vi "Poly-fit.vi"(3 "QPD signal (V)":dbl[](array[numeric]), 5 "stage position (um)":dbl[](array[numeric])) -> (1 "Polynomial Coefficients":dbl[](array[numeric]), 2 "Best stage position":dbl[](array[numeric]))   [LabVIEW 2014]
uses:
  <vilib>/Analysis/NI_AALPro.lvlib
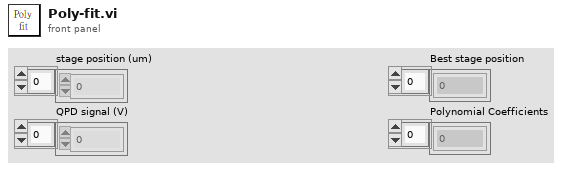
[diagram p1: front panel]
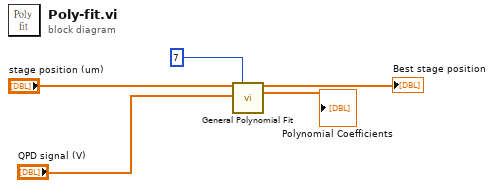
[diagram p0: block diagram]
diagram:
  n1 = call <vilib>:"General Polynomial Fit.vi"("Y"="stage position (um)", "polynomial order"=7, "X"="QPD signal (V)") -> ("Best Polynomial Fit"=→"Best stage position":dbl[], "Polynomial Coefficients"=→"Polynomial Coefficients":dbl[])  [unwired: 9 in, 2 out]
